vi "direction to travel.vi"(9 "current location":cluster{"x":i16, "y":i16}, 11 "rectangle object":T2) -> (2 "relative object data":T1)   [LabVIEW 2009]
uses:
  object.ctl
  object relations.ctl
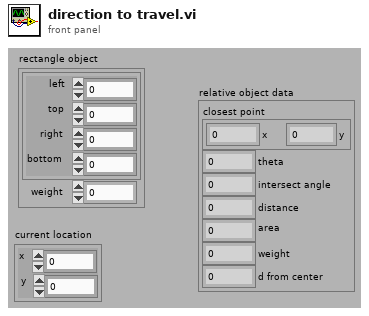
[diagram p1: front panel]
types:
  T1 = typedef "object relations.ctl" = cluster{"closest point":cluster{"x":i16, "y":i16}, "theta":sgl, "intersect angle":sgl, "distance":i16, "area":i16, "weight":sgl, "d from center":i16}
  T2 = typedef "object.ctl" = cluster{"rect":cluster{"left":i16, "top":i16, "right":i16, "bottom":i16}, "weight":sgl}
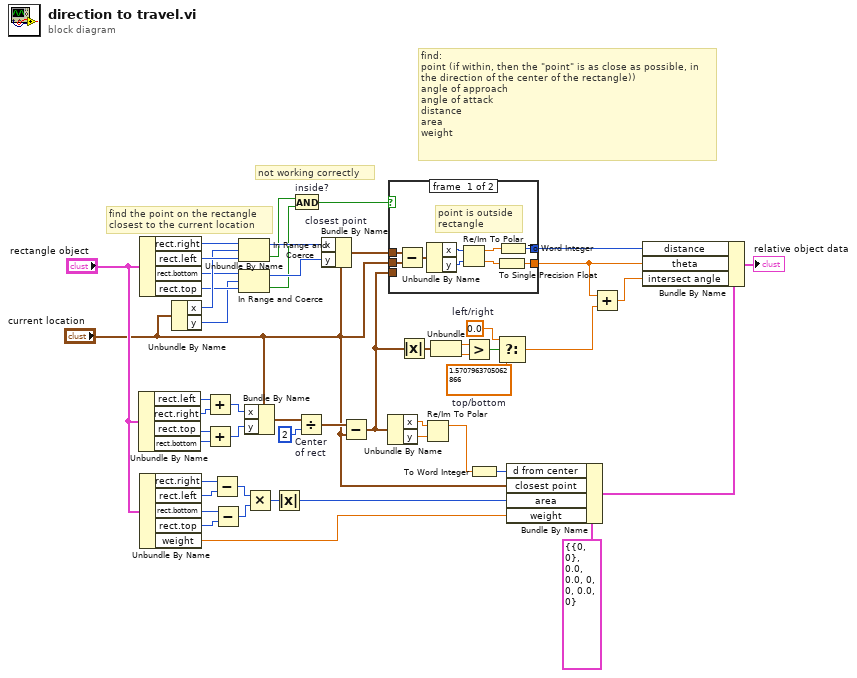
[diagram p0: block diagram]
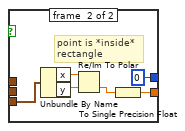
[diagram p2: hidden frame]
diagram:
  w23 = sgl 1.5707964  # top/bottom
  w24 = sgl 0.0  # left/right
  # "not working correctly"
  # "find the point on the rectangle\nclosest to the current location"
  # "find:\npoint (if within, then the \"point\" is as close as possible, in the direction of the center of the rectangle))\nangle of approach\nangle of attack\ndistance\narea\nweight"
  n1 = Unbundle By Name("rectangle object") -> ("rect.left"=w29:i16, "rect.right"=w30:i16, "rect.top"=w31:i16, "rect.bottom"=w32:i16)
  n2 = Unbundle By Name("rectangle object") -> ("rect.right"=w50:i16, "rect.left"=w49:i16, "rect.bottom"=w46:i16, "rect.top"=w47:i16)
  n3 = Unbundle By Name("rectangle object") -> ("rect.right"=w18:i16, "rect.left"=w17:i16, "rect.bottom"=w16:i16, "rect.top"=w15:i16, "weight"=w9:sgl)
  n4 = Unbundle By Name("current location") -> ("x"=w48:i16, "y"=w45:i16)
  n5 = Add(x=w29, y=w30) -> (x+y=w33:i16)
  n6 = Add(x=w31, y=w32) -> (x+y=w34:i16)
  n7 = Subtract(x=w18, y=w17) -> (x-y=w13:i16)
  n8 = Subtract(x=w16, y=w15) -> (x-y=w14:i16)
  n9 = In Range and Coerce(upper limit=w50, x=w48, lower limit=w49) -> (coerced(x)=w44:i16, In Range?=w41:bool)
  n10 = In Range and Coerce(upper limit=w46, x=w45, lower limit=w47) -> (coerced(x)=w43:i16, In Range?=w42:bool)
  n11 = Bundle By Name(cluster="current location", "x"=w33, "y"=w34) -> (w35:cluster{"x":i16, "y":i16})
  n12 = Multiply(x=w13, y=w14) -> (x*y=w10:i16)
  n13 = Absolute Value(x=w10) -> (abs(x)=w1:i16)
  n14 = And "inside?"(x=w41, y=w42) -> (x .and. y?=w40:bool)
  n15 = Divide "Center\nof rect"(x=w35, y=2) -> (x/y=w37:cluster{"x":dbl, "y":dbl})
  n16 = Bundle By Name "closest point"(cluster="current location", "x"=w44, "y"=w43) -> (w39:cluster{"x":i16, "y":i16})
  n17 = Subtract(x=w37, y="current location") -> (x-y=w4:cluster{"x":dbl, "y":dbl})
  n18 = Unbundle By Name(w4) -> ("x"=w5:dbl, "y"=w6:dbl)
  n19 = case shown="False" w40 {
    tunnel: w39 -> [w59 _]
    tunnel: "current location" -> [w58 _]
    tunnel: [w51 w60] -> w22
    tunnel: [w53 i16 0 ("distance")] -> w38
    tunnel: w4 -> [_ w61]
    frame #0 {
      # "point is outside\nrectangle"
      n20 = Subtract(x=w59, y=w58) -> (x-y=w57:cluster{"x":i16, "y":i16})
      n21 = Unbundle By Name(w57) -> ("x"=w56:i16, "y"=w55:i16)
      n22 = Re/Im To Polar(2:w55, 3:w56) -> (0:w52:dbl, 1:w54:dbl)
      n23 = To Single Precision Float(number=w52) -> (single precision float=w51:sgl)
      n24 = To Word Integer(number=w54) -> (16bit integer=w53:i16)
    }
    frame #1 {
      # "point is *inside*\nrectangle"
      n25 = Unbundle By Name(w61) -> ("x"=w65:dbl, "y"=w64:dbl)
      n26 = Re/Im To Polar(2:w64, 3:w65) -> (0:w63:dbl)  [unwired: 1 out]
      n27 = To Single Precision Float(number=w63) -> (single precision float=w60:sgl)
    }
  }
  n28 = Absolute Value(x=w4) -> (abs(x)=w27:cluster{"x":dbl, "y":dbl})
  n29 = Re/Im To Polar(2:w6, 3:w5) -> (1:w2:dbl)  [unwired: 1 out]
  n30 = Unbundle(w27) -> ("x"=w26:dbl, "y"=w25:dbl)
  n31 = Greater?(x=w26, y=w25) -> (0:w28:bool)
  n32 = To Word Integer(number=w2) -> (16bit integer=w3:i16)
  n33 = Select(t=w24, s=w28, f=w23) -> (s? t:f=w21:sgl)
  n34 = Bundle By Name(cluster=T1 {"closest point"={"x"=0, "y"=0}, "theta"=0.0, "intersect angle"=0.0, "distance"=0, "area"=0, "weight"=0.0, "d from center"=0} ("Object relations"), "d from center"=w3, "closest point"="current location", "area"=w1, "weight"=w9) -> (w8:T1)
  n35 = Add(x=w22, y=w21) -> (x+y=w20:sgl)
  n36 = Bundle By Name(cluster=w8, "distance"=w38, "theta"=w22, "intersect angle"=w20) -> (→"relative object data":T1)
